vi "sendMessage.vi"(8 "error in (no error)":errorcluster, 9 "data":variant, 10 "message":string, 11 "MsgUETaskChannel in":refnum<class "MsgQueueTaskChannel.lvclass">) -> (0 "error out":errorcluster, 3 "MsgUETaskChannel out":refnum<class "MsgQueueTaskChannel.lvclass">)   [LabVIEW 2023, in "TLC_Daemon.lvlib" / "MsgQueueTaskChannel.lvclass"]
uses:
  MsgQueueTaskChannel.lvclass
  Ctrls/msg.ctl
  MsgQueueTaskChannel.lvclass/MsgQueueTaskChannel.ctl
  TLC_Daemon.lvlib
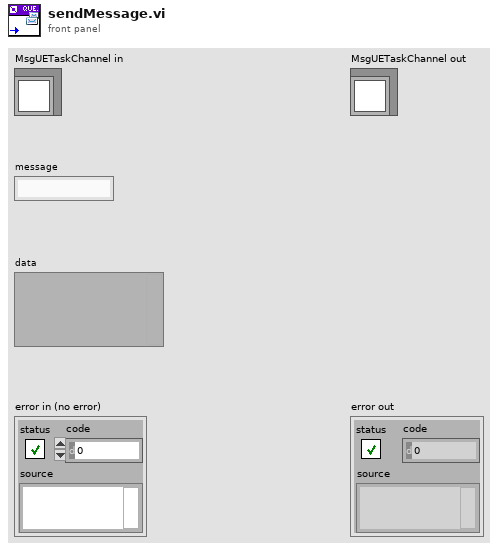
[diagram p1: front panel]
types:
  T1 = typedef "TLC_Daemon.lvlib/msg.ctl" = cluster{"message":string, "data":variant}
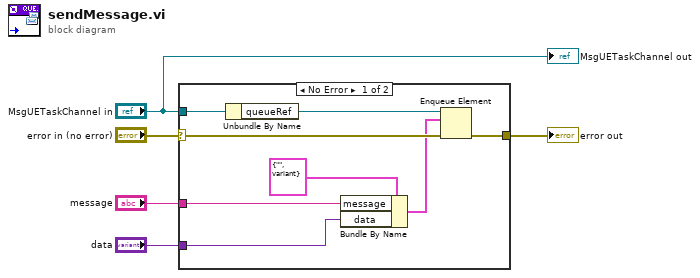
[diagram p0: block diagram]
diagram:
  n1 = case shown="No Error" "error in (no error)" {
    selector: "error in (no error)" -> [w10 w14]
    tunnel: [w11 w14] -> w4
    tunnel: "MsgUETaskChannel in" -> [w13 _]
    tunnel: "message" -> [w8 _]
    tunnel: "data" -> [w7 _]
    frame No Error {
      n2 = Unbundle By Name(w13) -> ("queueRef"=w12:refnum<queue>)
      n3 = Bundle By Name(cluster=T1 {"message"="", "data"=variant} ("event data"), "message"=w8, "data"=w7) -> (w6:T1)
      n4 = Enqueue Element(queue=w12, element=w6, error in (no error)=w10) -> (error out=w11:errorcluster)  [unwired: 1 in, 2 out]
    }
    frame Error {
    }
  }
  "error out" <- w4
  "MsgUETaskChannel out" <- "MsgUETaskChannel in"
